vi "Async Stream ReadDI.vi"(8 "error in (no error)":errorcluster, 11 "DIOSessions In":T1={"Array of DI Sessions"=[], "Array of DO Sessions"=[], "Stream ReadDI"={"gRPCid ReadDI"=0, "DISessionName"="", "Stream Status ReadDI"=FALSE, "Async Stop ReadDI Queue"=refnum, "DI Task"="", "ms to wait"=500}}) -> (0 "error out":errorcluster)   [LabVIEW 2019, in "ctet_dio_User Library.lvlib"]
uses:
  ctet_dio_User Library.lvlib
  Types/DIOSessions.ctl
  Types/DISession.ctl
  Types/DOSession.ctl
  Types/StreamReadDI.ctl
  Servers/ctet_dio/gRPC lvSupport/Server API/typeDefs/grpcId.ctl
  Servers/ctet_dio/ctet_dio Class/RPC Messages/measurementservice_ErrorOut/measurementservice_ErrorOut_Data.ctl
  Servers/ctet_dio/ctet_dio Class/RPC Messages/measurementservice_ReadDIResponse/measurementservice_ReadDIResponse_Data.ctl
  <vilib>/DAQmx/read.llb/DAQmx Read (Digital 1D Bool 1Chan 1Samp).vi
  <vilib>/DAQmx/read.llb/DAQmx Read (Digital 1D Bool NChan 1Samp 1Line).vi
  <vilib>/DAQmx/miscellaneous.llb/DAQmx Fill In Error Info.vi
  Servers/ctet_dio/ctet_dio Class/ctet_dio.lvclass
  Servers/ctet_dio/gRPC lvSupport/gprc-lvsupport.lvlib
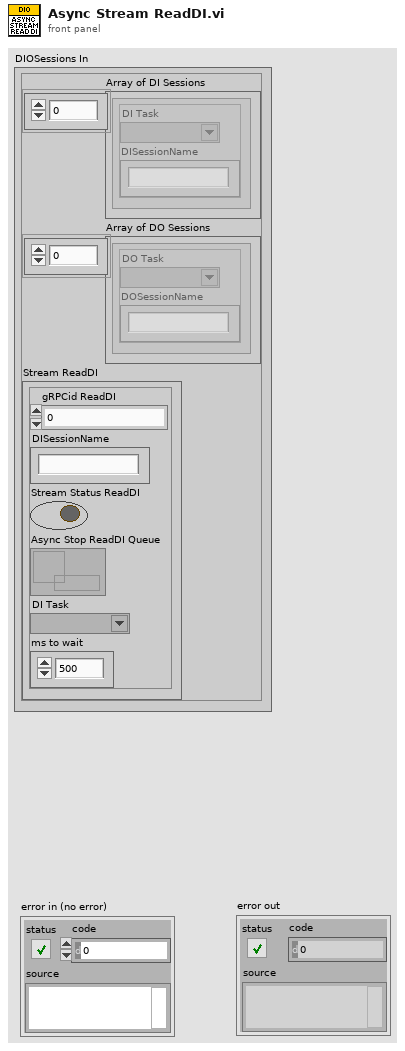
[diagram p1: front panel]
types:
  T1 = typedef "ctet_dio_User Library.lvlib/DIOSessions.ctl" = cluster{"Array of DI Sessions":T2[], "Array of DO Sessions":T3[], "Stream ReadDI":T4}
  T2 = typedef "ctet_dio_User Library.lvlib/DISession.ctl" = cluster{"DI Task":refnum<k21>, "DISessionName":string}
  T3 = typedef "ctet_dio_User Library.lvlib/DOSession.ctl" = cluster{"DO Task":refnum<k21>, "DOSessionName":string}
  T4 = typedef "ctet_dio_User Library.lvlib/StreamReadDI.ctl" = cluster{"gRPCid ReadDI":T5, "DISessionName":string, "Stream Status ReadDI":bool, "Async Stop ReadDI Queue":refnum<queue>, "DI Task":refnum<k21>, "ms to wait":u32}
  T5 = typedef "ctet_dio.lvlib/gprc-lvsupport.lvlib/grpcId.ctl" = u64
  T6 = typedef "ctet_dio.lvlib/ctet_dio.lvclass/measurementservice_ReadDIResponse_Data.ctl" = cluster{"DISessionName":string, "DIData":bool[], "error":T7}
  T7 = typedef "ctet_dio.lvlib/ctet_dio.lvclass/measurementservice_ErrorOut_Data.ctl" = cluster{"errCode":i64, "errMessage":string}
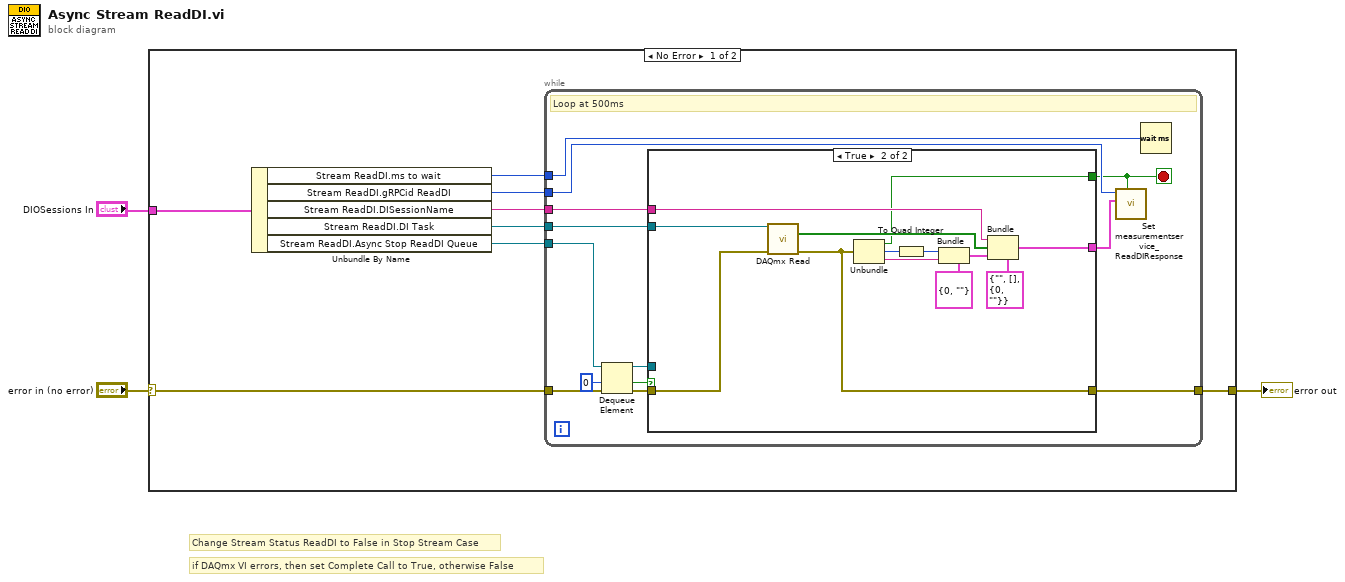
[diagram p0: block diagram]
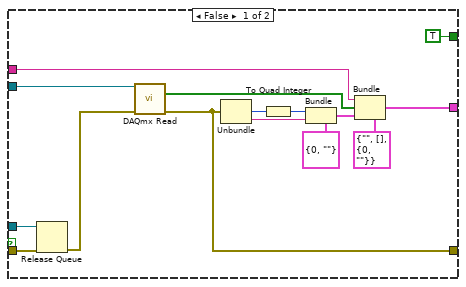
[diagram p2: hidden frame]
diagram:
  # "if DAQmx VI errors, then set Complete Call to True, otherwise False"
  # "Change Stream Status ReadDI to False in Stop Stream Case"
  n1 = case shown="No Error" "error in (no error)" {
    selector: "error in (no error)" -> [w8 w53]
    tunnel: [w5 w53] -> w3
    tunnel: "DIOSessions In" -> [w11 _]
    frame No Error {
      n2 = Unbundle By Name(w11) -> ("Stream ReadDI.ms to wait"=w4:u32, "Stream ReadDI.gRPCid ReadDI"=w10:T5, "Stream ReadDI.DISessionName"=w7:string, "Stream ReadDI.DI Task"=w9:refnum<k21>, "Stream ReadDI.Async Stop ReadDI Queue"=w6:refnum<queue>)
      n3 = while {
        tunnel: w10 -> [w15]
        tunnel: w9 -> [w24]
        tunnel: w8 -> [w21]
        tunnel: w7 -> [w23]
        tunnel: w6 -> [w22]
        tunnel: [w14] -> w5
        tunnel: w4 -> [w12]
        stop <- w13 stop-if-true
        # "Loop at 500ms"
        n4 = Dequeue Element(queue=w22, timeout in ms (-1)=0, error in (no error)=w21) -> (queue out=w18:refnum<queue>, timed out?=w19:bool, error out=w17:errorcluster)  [unwired: 1 out]
        n5 = case shown="True" w19 {
          tunnel: w24 -> [w29 w45]
          tunnel: w23 -> [w25 w44]
          tunnel: w18 -> [w39 _]
          tunnel: w17 -> [w38 w41]
          tunnel: [w26 w43] -> w16
          tunnel: [TRUE ("Complete Call (T)") w40] -> w13
          tunnel: [w27 w42] -> w14
          frame False {
            n6 = Release Queue(queue=w39, error in (no error)=w38) -> (error out=w28:errorcluster)  [unwired: 1 in, 2 out]
            n7 = call-poly <vilib>:"DAQmx Read.vi"("task/channels in"=w29, "error in"=w28) -> ("data"=w30:bool[], "error out"=w27:errorcluster)  [unwired: 11 in, 1 out]
            n8 = Unbundle(w27) -> ("code"=w34:i32, "source"=w35:string)  [unwired: 1 out]
            n9 = To Quad Integer(1:w34) -> (0:w33:i64)
            n10 = Bundle(cluster=T7 {"errCode"=0, "errMessage"=""} ("error"), "errCode"=w33, "errMessage"=w35) -> (w31:T7)
            n11 = Bundle(cluster=T6 {"DISessionName"="", "DIData"=[], "error"={"errCode"=0, "errMessage"=""}} ("measurementservice_ReadDIResponse_Data"), "DISessionName"=w25, "DIData"=w30, "error"=w31) -> (w26:T6)
          }
          frame True {
            n12 = call-poly <vilib>:"DAQmx Read.vi"("task/channels in"=w45, "error in"=w41) -> ("data"=w46:bool[], "error out"=w42:errorcluster)  [unwired: 11 in, 1 out]
            n13 = Unbundle(w42) -> ("status"=w40:bool, "code"=w50:i32, "source"=w51:string)
            n14 = To Quad Integer(1:w50) -> (0:w49:i64)
            n15 = Bundle(cluster=T7 {"errCode"=0, "errMessage"=""} ("error"), "errCode"=w49, "errMessage"=w51) -> (w47:T7)
            n16 = Bundle(cluster=T6 {"DISessionName"="", "DIData"=[], "error"={"errCode"=0, "errMessage"=""}} ("measurementservice_ReadDIResponse_Data"), "DISessionName"=w44, "DIData"=w46, "error"=w47) -> (w43:T6)
          }
        }
        n17 = call "Set measurementservice_ReadDIResponse.vi"("Complete Call (T)"=w13, "Message Data"=w16, "gRPCid"=w15) -> ()  [unwired: 8 in, 1 out]
        n18 = Wait (ms)(milliseconds to wait=w12) -> ()  [unwired: 1 out]
      }
    }
    frame Error {
    }
  }
  "error out" <- w3
